vi "getAttribute.vi"(0 "HGF_IMAQDevice":refnum<class "HGF_IMAQDevice.lvclass">, 1 "Attribute Name":string, 5 "error in (no error)":errorcluster) -> (14 "dup HGF_IMAQDevice":refnum<class "HGF_IMAQDevice.lvclass">, 15 "IMAQ Attribute":variant, 19 "error out":errorcluster)   [LabVIEW 2014, in "HGF_IMAQ.lvlib" / "HGF_IMAQDevice.lvclass"]
doc: "Return the name of camera."
uses:
  HGF_IMAQDevice.lvclass
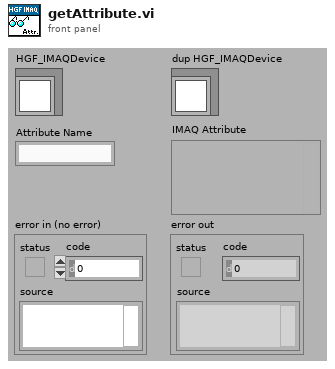
[diagram p1: front panel]
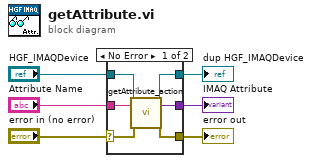
[diagram p0: block diagram]
diagram:
  n1 = case shown="No Error" "error in (no error)" {
    selector: "error in (no error)" -> [w12 w13]
    tunnel: [w11 w13] -> w5
    tunnel: [w8 w14] -> w3
    tunnel: "HGF_IMAQDevice" -> [w9 w14]
    tunnel: "Attribute Name" -> [w10 _]
    tunnel: [w7 _] -> w1
    frame No Error {
      n2 = call-dynamic "getAttribute_action.vi"("HGF_IMAQDevice"=w9, "Attribute Name"=w10, "error in (no error)"=w12) -> ("dup HGF_IMAQDevice"=w8:refnum<class "HGF_IMAQDevice.lvclass">, "IMAQ Attribute"=w7:variant, "error out"=w11:errorcluster)  [unwired: 14 in]
    }
    frame Error {
    }
  }
  "error out" <- w5
  "dup HGF_IMAQDevice" <- w3
  "IMAQ Attribute" <- w1
